vi "Read tau Obs.vi"(8 "error in (no error)":errorcluster, 11 "tCRD in":refnum<class "tCRD.lvclass">) -> (0 "error out":errorcluster, 2 "tauObs":refnum<class "File Observer.lvclass">, 3 "tCRD out":refnum<class "tCRD.lvclass">)   [LabVIEW 2015, in "tCRD.lvclass"]
uses:
  tCRD.lvclass
  Reusable/File IO/Class/File Observer.lvclass
  tCRD.lvclass/tCRD.ctl
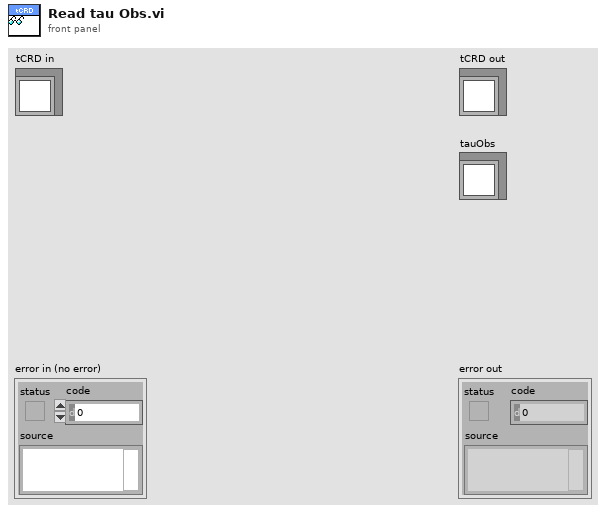
[diagram p1: front panel]
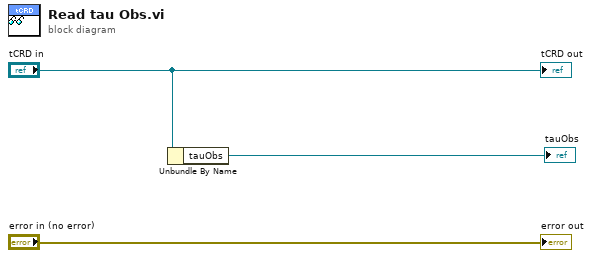
[diagram p0: block diagram]
diagram:
  n1 = Unbundle By Name("tCRD in") -> ("tauObs"=→"tauObs":refnum<class "File Observer.lvclass">)
  "error out" <- "error in (no error)"
  "tCRD out" <- "tCRD in"
